vi "SIM Let ZC Adjust Proposed StepSize.vi"(4 "current timestep base":dbl, 5 "proposed step time":dbl, 6 "proposed step size":dbl, 7 "max step ratio":dbl) -> (2 "proposed step size out":dbl, 3 "max step ratio out":dbl)   [LabVIEW 2017]
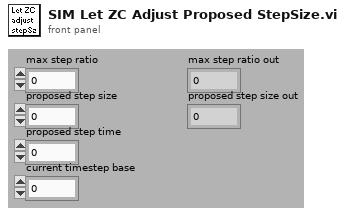
[diagram p1: front panel]
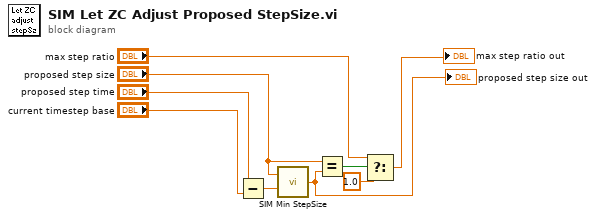
[diagram p0: block diagram]
diagram:
  n1 = Subtract(x="proposed step time", y="current timestep base") -> (x-y=w9:dbl)
  n2 = call <vilib>:"SIM Min StepSize.vi"("step size 2"=w9, "step size 1"="proposed step size") -> ("min step size"=w6:dbl)
  "proposed step size out" <- w6
  n3 = Equal?(x="proposed step size", y=w6) -> (x = y?=w8:bool)
  n4 = Select(t="max step ratio", s=w8, f=1.0) -> (s? t:f=→"max step ratio out":dbl)
